vi "circular buffer handler.vi"(0 "StreamToWrite":u8[](array[numeric]), 7 "ByteToWrite":u8, 11 "NumberOfBytes":i32, 13 "Enum":T1(ring)) -> (4 "OutputBytes":u8[](array[numeric]), 8 "OK":bool, 15 "Output":i32)   [LabVIEW 2010]
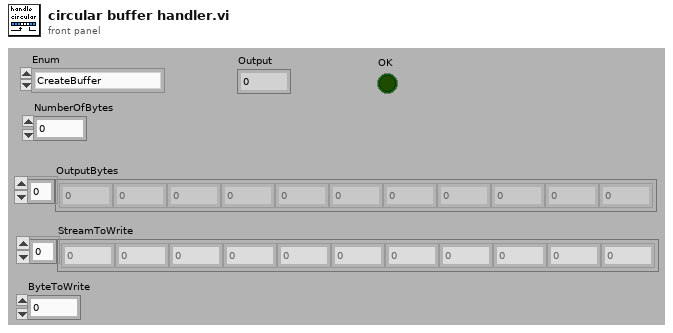
[diagram p1: front panel]
types:
  T1 = enum16{"CreateBuffer", "WriteBytes", "WriteByte", "AvailableMemory", "OccupiedMemory", "CheckBytes", "ReadBytes"}
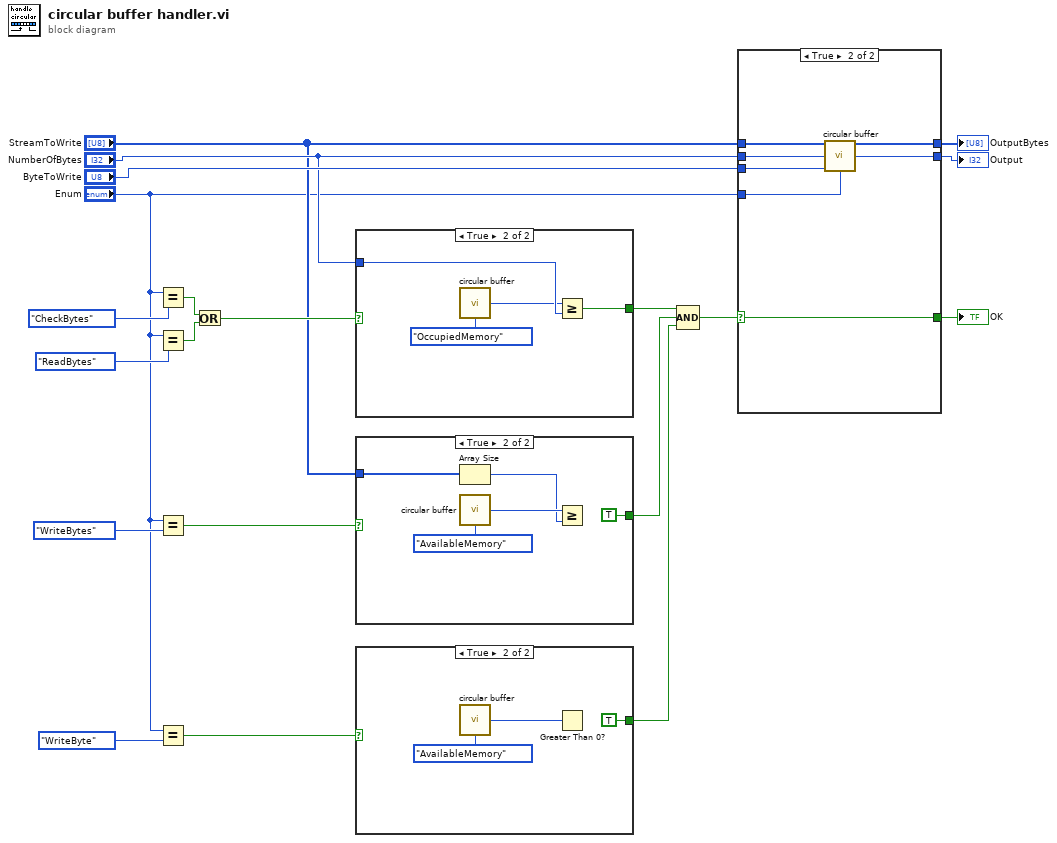
[diagram p0: block diagram]
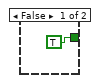
[diagram p2: hidden frame]
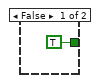
[diagram p3: hidden frame]
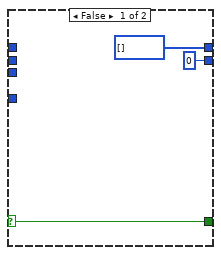
[diagram p4: hidden frame]
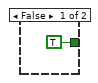
[diagram p5: hidden frame]
diagram:
  n1 = Equal?(x="Enum", y=T1."CheckBytes") -> (x = y?=w14:bool)
  n2 = Equal?(x="Enum", y=T1."ReadBytes") -> (x = y?=w15:bool)
  n3 = Equal?(x="Enum", y=T1."WriteBytes") -> (x = y?=w10:bool)
  n4 = Equal?(x="Enum", y=T1."WriteByte") -> (x = y?=w8:bool)
  n5 = Or(x=w14, y=w15) -> (x .or. y?=w13:bool)
  n6 = case shown="True" w13 {
    tunnel: "NumberOfBytes" -> [_ w24]
    tunnel: [TRUE w22] -> w6
    frame False {
    }
    frame True {
      n7 = call "circular buffer.vi"("Enum"=T1."OccupiedMemory") -> ("Output"=w23:i32)  [unwired: 13 in, 1 out]
      n8 = Greater Or Equal?(x=w23, y=w24) -> (x >= y?=w22:bool)
    }
  }
  n9 = case shown="True" w10 {
    tunnel: [TRUE TRUE] -> w5
    tunnel: "StreamToWrite" -> [_ w30]
    frame False {
    }
    frame True {
      n10 = Array Size(array=w30) -> (size(s)=w28:i32)
      n11 = call "circular buffer.vi"("Enum"=T1."AvailableMemory") -> ("Output"=w29:i32)  [unwired: 13 in, 1 out]
      n12 = Greater Or Equal?(x=w29, y=w28) -> ()  [unwired: 1 out]
    }
  }
  n13 = case shown="True" w8 {
    tunnel: [TRUE TRUE] -> w4
    frame False {
    }
    frame True {
      n14 = call "circular buffer.vi"("Enum"=T1."AvailableMemory") -> ("Output"=w34:i32)  [unwired: 13 in, 1 out]
      n15 = Greater Than 0?(x=w34) -> ()  [unwired: 1 out]
    }
  }
  n16 = Compound Arithmetic op=AND(w6, w5, w4) -> (w3:bool)
  n17 = case shown="True" w3 {
    selector: w3 -> [w38 w40]
    tunnel: "StreamToWrite" -> [_ w45]
    tunnel: "ByteToWrite" -> [_ w44]
    tunnel: [u8[] [] ("OutputBytes") w43] -> w19
    tunnel: [0 ("Output") w42] -> w18
    tunnel: "NumberOfBytes" -> [_ w41]
    tunnel: [w38 w40] -> w2
    tunnel: "Enum" -> [_ w39]
    frame False {
    }
    frame True {
      n18 = call "circular buffer.vi"("StreamToWrite"=w45, "NumberOfBytes"=w41, "ByteToWrite"=w44, "Enum"=w39) -> ("OutputBytes"=w43:u8[], "Output"=w42:i32)  [unwired: 10 in]
    }
  }
  "Output" <- w18
  "OutputBytes" <- w19
  "OK" <- w2
